vi "Change SubPanelPosition.vi"(8 "error in (no error)":errorcluster, 9 "NewBnds":T1, 10 "SubPnl Refnum":refnum<vi>, 11 "MainUI in":refnum<class "UI_Top_Customer.lvclass">) -> (0 "error out":errorcluster, 3 "MainUI out":refnum<class "UI_Top_Customer.lvclass">)   [LabVIEW 2021, in "UI_Top_Customer.lvclass"]
uses:
  UI_Top_Customer.lvclass
  <vilib>/Utility/miscctls.llb/LVRectTypeDef.ctl
  UI_Top_Customer.lvclass/UI_Top_Customer.ctl
panel:
  in  "y":i16=200
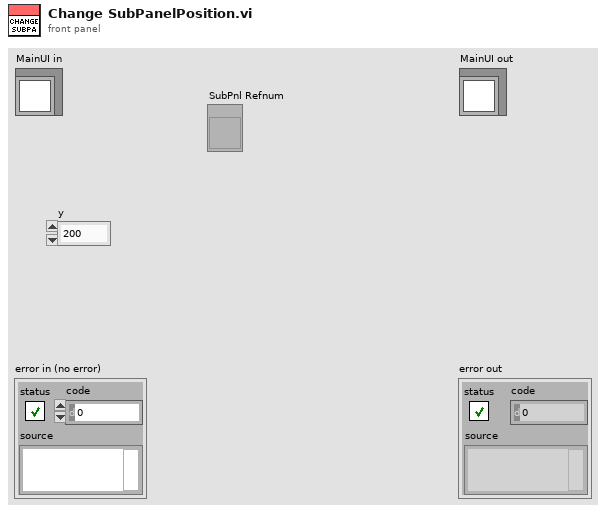
[diagram p1: front panel]
types:
  T1 = typedef "LVRectTypeDef.ctl" = cluster{"Left":i16, "Top":i16, "Right":i16, "Bottom":i16}
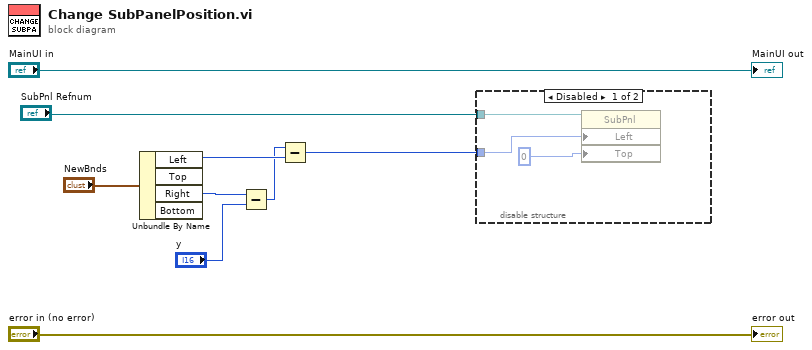
[diagram p0: block diagram]
diagram:
  n1 = Unbundle By Name("NewBnds") -> ("Left"=w6:i16, "Right"=w4:i16)  [unwired: 2 out]
  n2 = Subtract(x=w4, y="y") -> (x-y=w1:i16)
  n3 = Subtract(x=w1, y=w6) -> (x-y=w2:i16)
  n4 = disable-structure shown="Disabled" {
    disable-tunnel: "SubPnl Refnum" -> [w12 _]
    disable-tunnel: w2 -> [w11 _]
    frame Disabled {
      n5 = property class="SubPnl"(reference=w12, "Left"=w11, "Top"=0 ("Position:Top")) -> ()  [unwired: 1 in, 2 out]
    }
    frame Enabled {
    }
  }
  "error out" <- "error in (no error)"
  "MainUI out" <- "MainUI in"
